vi "SENS_COUP_ALL_NONE.vi"(0 "VISA IN":refnum<visa-resource-name>, 1 "Sweep Mode(ALL or NONE)":string(combo)="NONE", 5 "error in":errorcluster, 7 "Channel":i32) -> (14 "VISA Out":refnum<visa-resource-name>, 19 "error out":errorcluster)   [LabVIEW 2018, in "PNA-X.lvlib"]
doc: "SENSe<cnum>:COUPle <ALL | NONE> \n(Read-Write) Sets the sweep mode as Chopped or Alternate. \nLearn about Alternate Sweep \nParameters \n<cnum> Any existing channel number; if unspecified, value is set to 1. \n<ALL | NONE> ALL - Sweep mode set to Chopped - reflection and transmission measured on \nthe same sweep. \nNONE - Sweep mode set to Alternate - reflection and transmission measured \non separate sweeps. Improves Mixer bounce and Isolation measurements. \nIncreases sweep time \nExamples SENS:COUP ALL \nsense2:couple none \nQuery Syntax SENSe<cnum>:COUPle? \nReturn Type Character \nDefault ALL"
uses:
  PNA-X.lvlib
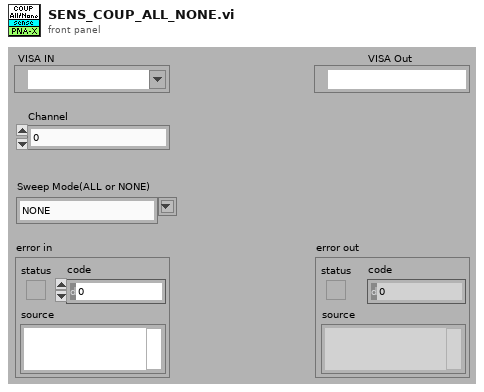
[diagram p1: front panel]
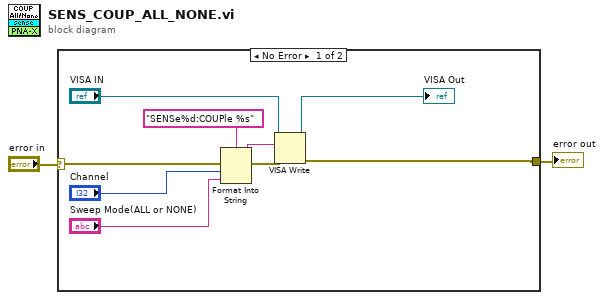
[diagram p0: block diagram]
diagram:
  n1 = case shown="No Error" "error in" {
    selector: "error in" -> [w11 w12]
    tunnel: [w6 w12] -> w1
    frame No Error {
      n2 = Format Into String(format string="SENSe%d:COUPle %s" ("Cmdline"), error in=w11, "Channel", "Sweep Mode(ALL or NONE)") -> (resulting string=w9:string, error out=w10:errorcluster)  [unwired: 1 in]
      n3 = VISA Write(VISA resource name="VISA IN", write buffer=w9, error in (no error)=w10) -> (VISA resource name out=→"VISA Out":refnum<visa-resource-name>, error out=w6:errorcluster)  [unwired: 1 out]
    }
    frame Error {
    }
  }
  "error out" <- w1
